vi "全局变量发送数据.vi"() -> ()   [LabVIEW 2010]
uses:
  传递波形全局变量.vi
panel:
  out "波形图表":dbl(graph)
  in  "延时":i16(slide)=100 min=0 max=200 step=10 scale=0.0..200.0
  in  "停止":bool
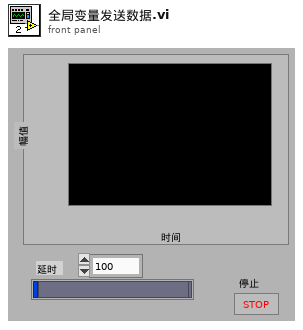
[diagram p1: front panel]
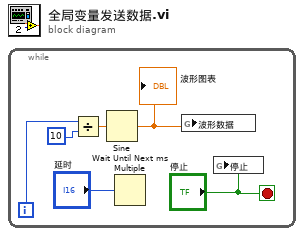
[diagram p0: block diagram]
diagram:
  n1 = while {
    i -> [w5]
    stop <- "停止" stop-if-true
    n2 = Divide(x=w5, y=10) -> (x/y=w3:dbl)
    n3 = Sine(x=w3) -> (sin(x)=w2:dbl)
    "波形图表" <- w2
    n4 = Wait Until Next ms Multiple(millisecond multiple="延时") -> ()  [unwired: 1 out]
    n5 = global write "传递波形全局变量.vi" "波形数据"(w2) -> ()
    n6 = global write "传递波形全局变量.vi" "停止"("停止") -> ()
  }
